vi "Error Log File.vi"(8 "error in":errorcluster, 9 "Write":string, 10 "File Options":T1=enum."Read File", 11 "File Name":string) -> (0 "error out":errorcluster, 1 "Read":string)   [LabVIEW 2023, in "HardwareAbstractionLayer_LVOOP.lvlib" / "Error Handler.lvclass"]
uses:
  Error Handler.lvclass
  Control/Error File.ctl
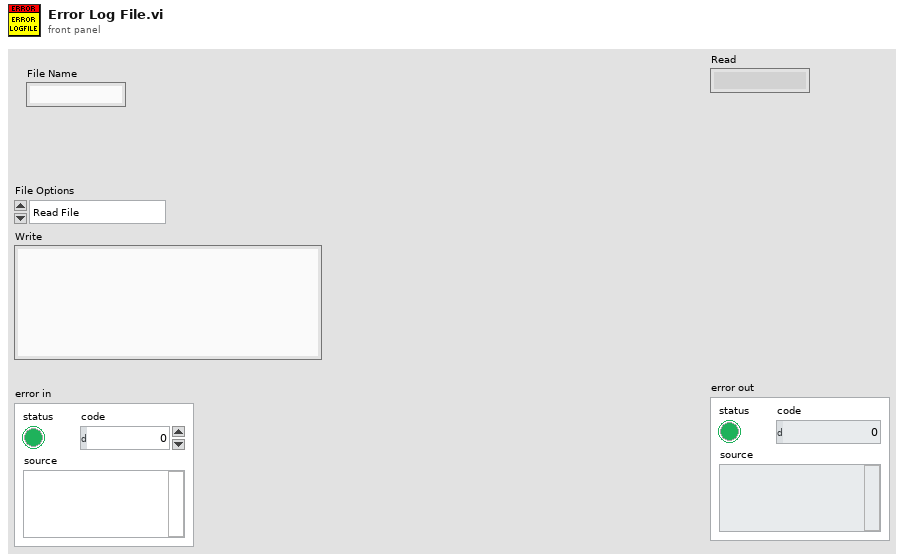
[diagram p1: front panel]
types:
  T1 = typedef "HardwareAbstractionLayer_LVOOP.lvlib/Error Handler.lvclass/Error File.ctl" = enum16{"Open", "Read File", "Write File", "Close"}
  T2 = enum16{"open", "replace", "create", "open or create", "replace or create", "replace or create with confirmation"}
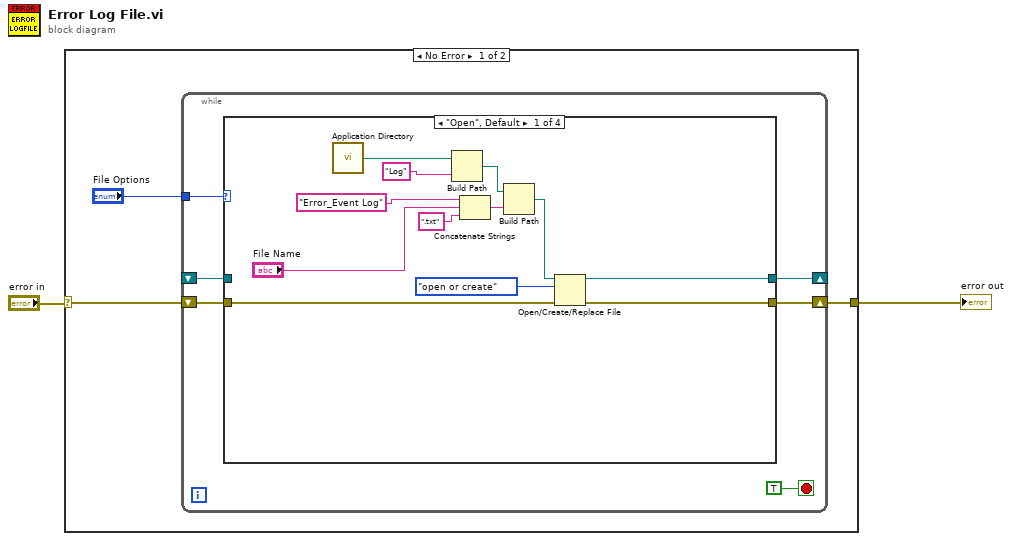
[diagram p0: block diagram]
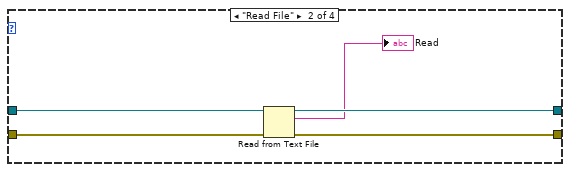
[diagram p2: hidden frame]
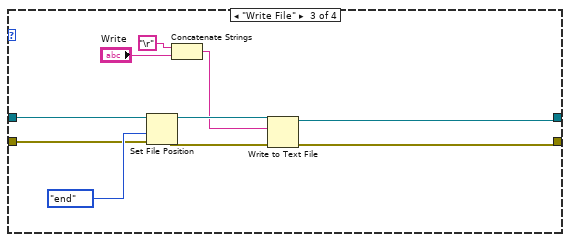
[diagram p3: hidden frame]
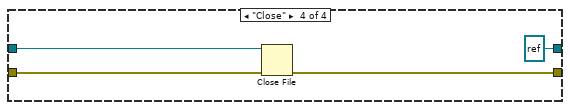
[diagram p4: hidden frame]
diagram:
  n1 = case shown="No Error" "error in" {
    selector: "error in" -> [w4 w43]
    tunnel: [w3 w43] -> w1
    frame No Error {
      n2 = while {
        tunnel: "File Options" -> [w11]
        shift-right: [w7] -> _
        shift-left: _ -> [w10]
        shift-right: [w8] -> w3
        shift-left: w4 -> [w9]
        stop <- TRUE stop-if-true
        n3 = case shown="\"Open\", Default" w11 {
          tunnel: w10 -> [_ w28 w33 w40]
          tunnel: w9 -> [w14 w27 w34 w42]
          tunnel: [w13 w26 w38 w41] -> w8
          tunnel: [w12 w25 w37 refnum<file> refnum ("refnum out")] -> w7
          frame "Open", Default {
            n4 = call <vilib>:"Application Directory.vi"() -> ("Application Directory"=w15:path)
            n5 = Build Path(base path=w15, name or relative path="Log") -> (appended path=w16:path)
            n6 = Concatenate Strings("Error_Event Log", "File Name", ".txt" ("string")) -> (w20:string)
            n7 = Build Path(base path=w16, name or relative path=w20) -> (appended path=w22:path)
            n8 = Open/Create/Replace File(file path (use dialog)=w22, error in=w14, operation (0:open)=T2."open or create") -> (refnum out=w12:refnum<file>, error out=w13:errorcluster)  [unwired: 3 in, 1 out]
          }
          frame "Read File" {
            n9 = Read from Text File(file (use dialog)=w28, error in=w27) -> (refnum out=w25:refnum<file>, text=→"Read":string, error out=w26:errorcluster)  [unwired: 2 in, 1 out]
          }
          frame "Write File" {
            n10 = Set File Position(refnum=w33, from (0:start)=enum16{"start", "end", "current"}."end", error in=w34) -> (refnum out=w32:refnum<file>, error out=w31:errorcluster)  [unwired: 1 in]
            n11 = Concatenate Strings("\r", "Write") -> (w30:string)
            n12 = Write to Text File(file (use dialog)=w32, text=w30, error in=w31) -> (refnum out=w37:refnum<file>, error out=w38:errorcluster)  [unwired: 1 in, 1 out]
          }
          frame "Close" {
            n13 = Close File(refnum=w40, error in=w42) -> (error out=w41:errorcluster)  [unwired: 1 out]
          }
        }
      }
    }
    frame Error {
    }
  }
  "error out" <- w1
